vi "9211_UI.vi"(8 "error in (no error)":errorcluster, 11 "Node Ptr":T1 format="%.0x") -> (0 "error out":errorcluster)   [LabVIEW 2019, in "Modules.lvlib" / "9211.lvclass"]
uses:
  9211.lvclass
  <vilib>/NI VeriStand/Custom Device API/Custom Device Item Ref.ctl
  RSI Module/SubPanel Command.ctl
  C:/Users/nitest/Desktop/Git 2019/niveristand-scan-engine-module-libraries/Source/RSI Module/RSI Module.lvclass
  9211.lvclass/9211.ctl
  RSI Module/RSI Module.lvclass
  <vilib>/NI VeriStand/Custom Device API/Custom Device API.lvlib
panel:
  out "_TCTypelabel":string="Thermocouple Type"
  out "_MeasUnitsLabel":string="Measurement Units" caption="MeasUnitsLabel"
  out "_Chan3Label":string="Channel 3"
  out "_Chan2Label":string="Channel 2"
  out "_Chan1Label":string="Channel 1"
  out "_Chan0Label":string="Channel 0"
  in  "Thermocouple Type 3":u8(ring) items=["J", "K", "T", "E", "R", "S", "N", "B"]
  in  "Thermocouple Type 2":u8(ring) items=["J", "K", "T", "E", "R", "S", "N", "B"]
  in  "Thermocouple Type 1":u8(ring) items=["J", "K", "T", "E", "R", "S", "N", "B"]
  in  "Thermocouple Type 0":u8(ring) items=["J", "K", "T", "E", "R", "S", "N", "B"]
  in  "Degree Range AI3":u8(ring)=2 items=["Raw Volts", "Degrees Kelvin", "Degrees Celsius", "Degrees Fahrenheit", "Degrees Rankine"]
  in  "Degree Range AI2":u8(ring)=2 items=["Raw Volts", "Degrees Kelvin", "Degrees Celsius", "Degrees Fahrenheit", "Degrees Rankine"]
  in  "Degree Range AI1":u8(ring)=2 items=["Raw Volts", "Degrees Kelvin", "Degrees Celsius", "Degrees Fahrenheit", "Degrees Rankine"]
  in  "Degree Range AI0":u8(ring)=2 items=["Raw Volts", "Degrees Kelvin", "Degrees Celsius", "Degrees Fahrenheit", "Degrees Rankine"]
  in  "SubPanel Event":refnum<user-event>
  in  "Header":cluster{"Section Name":string}={"Section Name"="NI 9205 Settings"}
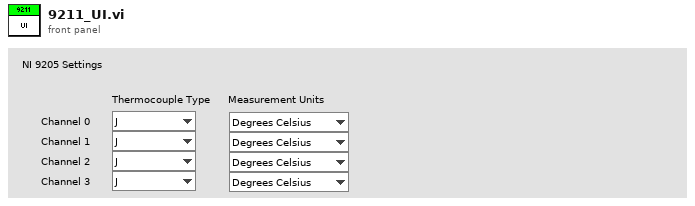
[diagram p1: front panel]
types:
  T1 = typedef "Custom Device API.lvlib/Custom Device Item Ref.ctl" = u64
  T2 = typedef "Modules.lvlib/RSI Module.lvclass/Module Models.ctl" = enum16{"Empty", "NI 9201", "NI 9203", "NI 9205", "NI 9206", "NI 9207", "NI 9208", "NI 9209", "NI 9210", "NI 9211", "NI 9212", "NI 9213", "NI 9214", "NI 9215", "NI 9216", "NI 9217", "NI 9219", "NI 9220", "NI 9221", "NI 9222", "NI 9223", "NI 9224", "NI 9225", "NI 9226", "NI 9227", "NI 9228", "NI 9229", "NI 9233", "NI 9234", "NI 9235", "NI 9236", "NI 9237", "NI 9239", "NI 9242", "NI 9244", "NI 9253", "NI 9263", "NI 9264", "NI 9265", "NI 9266", "NI 9269", "NI 9344", "NI 9350", "NI 9375", "NI 9401", "NI 9402", "NI 9403", "NI 9411", "NI 9421", "NI 9422", "NI 9423", "NI 9425", "NI 9426", "NI 9435", "NI 9436", "NI 9437", "NI 9472", "NI 9474", "NI 9475", "NI 9476", "NI 9477", "NI 9478", "NI 9481", "NI 9482", "NI 9485"}
  T3 = cluster{"Degree range":u32, "Thermocouple type":u32}[]
  T4 = cluster{"Degree range":u32, "Thermocouple type":u32}
  T5 = typedef "Modules.lvlib/RSI Module.lvclass/SubPanel Command.ctl" = enum16{"Stop"}
  T6 = cluster{"Degree Range AI0":u8, "Thermocouple Type 0":u8}
  T7 = cluster{"Degree Range AI1":u8, "Thermocouple Type 1":u8}
  T8 = cluster{"Degree Range AI2":u8, "Thermocouple Type 2":u8}
  T9 = cluster{"Degree Range AI3":u8, "Thermocouple Type 3":u8}
  T10 = cluster{"Degree Range AI3":u8, "Thermocouple Type 3":u8}[]
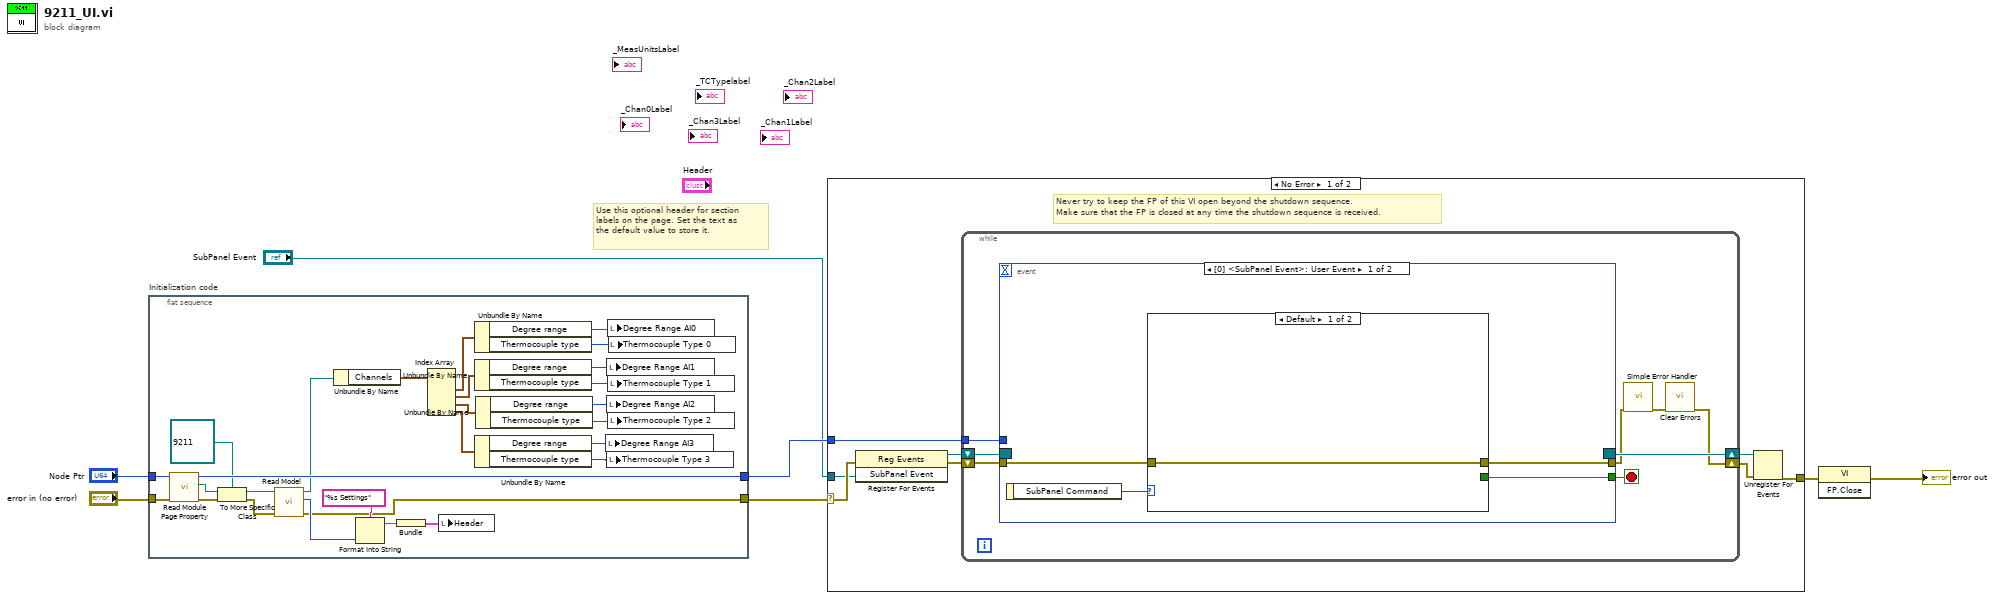
[diagram p0: block diagram]
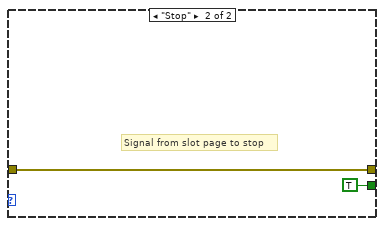
[diagram p2: hidden frame]
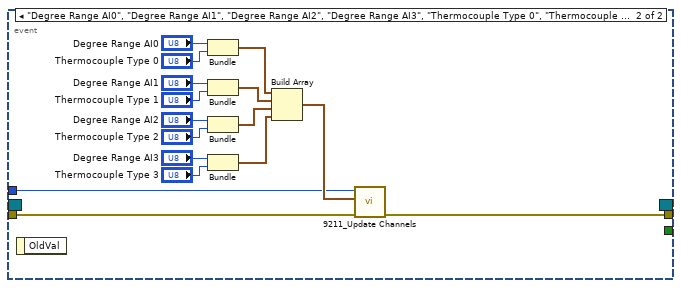
[diagram p3: hidden frame]
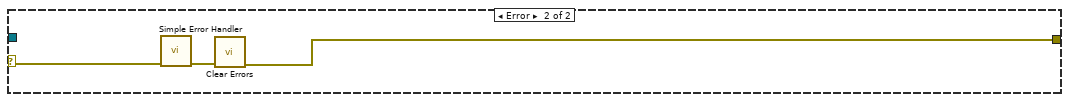
[diagram p4: hidden frame]
diagram:
  # "Use this optional header for section labels on the page. Set the text as the default value to store it."
  n1 = flat-sequence "Initialization code" {
    tunnel: "error in (no error)" -> [w33]
    tunnel: "Node Ptr" -> [w34]
    tunnel: [w21] -> w1
    tunnel: [w32] -> w4
    frame #0 {
      n2 = call "Read Module Page Property.vi"("error in (no error)"=w33, "Node Ptr In"=w34) -> ("error out"=w31:errorcluster, "RSI Module"=w29:refnum<class "RSI Module.lvclass">, "Node Ptr Out"=w32:T1)  [unwired: 7 in]
      n3 = To More Specific Class(target class=refnum<class "9211.lvclass"> refnum ("9205 in"), reference=w29, error in=w31) -> (specific class reference=w28:refnum<class "9211.lvclass">, error out=w27:errorcluster)
      n4 = call "Read Model.vi"("error in (no error)"=w27, "RSI Module in"=w28) -> ("error out"=w21:errorcluster, "Model"=w25:T2, "RSI Module out"=w22:refnum<class "9211.lvclass">)  [unwired: 7 in]
      n5 = Unbundle By Name(w22) -> ("Channels"=w20:T3)
      n6 = Format Into String(format string="%s Settings", w25) -> (resulting string=w23:string)  [unwired: 2 in, 1 out]
      n7 = Bundle(w23) -> (w26:cluster{string})  [unwired: 1 in]
      n8 = Index Array(array=w20) -> (element #1=w17:T4, element #2=w16:T4, element #3=w15:T4, element #4=w14:T4)  [unwired: 4 in]
      n9 = local write "Header"(w26) -> ()
      n10 = Unbundle By Name(w17) -> ("Degree range"=w19:u32, "Thermocouple type"=w18:u32)
      n11 = Unbundle By Name(w16) -> ("Degree range"=w13:u32, "Thermocouple type"=w12:u32)
      n12 = Unbundle By Name(w14) -> ("Degree range"=w9:u32, "Thermocouple type"=w8:u32)
      n13 = Unbundle By Name(w15) -> ("Degree range"=w11:u32, "Thermocouple type"=w10:u32)
      n14 = local write "Degree Range AI3"(w9) -> ()
      n15 = local write "Degree Range AI1"(w13) -> ()
      n16 = local write "Degree Range AI2"(w11) -> ()
      n17 = local write "Thermocouple Type 3"(w8) -> ()
      n18 = local write "Degree Range AI0"(w19) -> ()
      n19 = local write "Thermocouple Type 1"(w12) -> ()
      n20 = local write "Thermocouple Type 2"(w10) -> ()
      n21 = local write "Thermocouple Type 0"(w18) -> ()
    }
  }
  n22 = case shown="No Error" w1 {
    selector: w1 -> [w36 w76]
    tunnel: [w40 w74] -> w7
    tunnel: w4 -> [w37 _]
    tunnel: "SubPanel Event" -> [w35 _]
    frame No Error {
      # "Never try to keep the FP of this VI open beyond the shutdown sequence.\nMake sure that the FP is closed at any time the shutdown sequence is received."
      n23 = register-events(error in=w36, w35) -> (reference out=w38:refnum<event-registration>, error out=w39:errorcluster)  [unwired: 1 in]
      n24 = while {
        tunnel: w37 -> [w46]
        shift-right: [w43] -> w41
        shift-left: w39 -> [w49]
        shift-right: [w50] -> w42
        shift-left: w38 -> [w48]
        stop <- w47 stop-if-true
        n25 = event shown="[0] <SubPanel Event>: User Event" {
          selector: w48 -> [_ _]
          dyn-events: [_ _] -> w50
          timeout: _ -> [_ _]
          tunnel: w49 -> [w53 w60]
          tunnel: [w52 _] -> w47
          tunnel: [w51 w61] -> w45
          tunnel: w46 -> [_ w58]
          event User Event {
            n26 = event-data() -> ("SubPanel Command"=w54:T5)  [unwired: 1 out]
            n27 = case shown="Default" w54 {
              tunnel: w53 -> [w55 w56]
              tunnel: [w55 w56] -> w51
              tunnel: [_ TRUE] -> w52
              frame Default {
              }
              frame "Stop" {
                # "Signal from slot page to stop"
              }
            }
          }
          event "Degree Range AI0", "Degree Range AI1", "Degree Range AI2", "Degree Range AI3", "Thermocouple Type 0", "Thermocouple Type 1", "Thermocouple Type 2", "Thermocouple Type 3": Value Change {
            n28 = event-data() -> ()  [unwired: 2 out]
            n29 = Bundle("Degree Range AI0"="Degree Range AI0", "Thermocouple Type 0"="Thermocouple Type 0") -> (w71:T6)  [unwired: 1 in]
            n30 = Bundle("Degree Range AI1"="Degree Range AI1", "Thermocouple Type 1"="Thermocouple Type 1") -> (w64:T7)  [unwired: 1 in]
            n31 = Bundle("Degree Range AI2"="Degree Range AI2", "Thermocouple Type 2"="Thermocouple Type 2") -> (w63:T8)  [unwired: 1 in]
            n32 = Bundle("Degree Range AI3"="Degree Range AI3", "Thermocouple Type 3"="Thermocouple Type 3") -> (w62:T9)  [unwired: 1 in]
            n33 = Build Array(w71, w64, w63, w62) -> (w59:T10)
            n34 = call "9211_Update Channels.vi"("error in"=w60, "Channels"=w59, "Node Ptr in"=w58) -> ("error out"=w61:errorcluster)  [unwired: 7 in, 1 out]
          }
        }
        n35 = call <vilib>:"Simple Error Handler.vi"("error in (no error)"=w45) -> ("error out"=w44:errorcluster)  [unwired: 1 in, 7 out]
        n36 = call <vilib>:"Clear Errors.vi"("error in (no error)"=w44) -> ("error out"=w43:errorcluster)  [unwired: 1 in, 5 out]
      }
      n37 = Unregister For Events(event registration refnum=w42, error in=w41) -> (error out=w40:errorcluster)
    }
    frame Error {
      n38 = call <vilib>:"Simple Error Handler.vi"("error in (no error)"=w76) -> ("error out"=w75:errorcluster)  [unwired: 1 in, 7 out]
      n39 = call <vilib>:"Clear Errors.vi"("error in (no error)"=w75) -> ("error out"=w74:errorcluster)  [unwired: 1 in, 5 out]
    }
  }
  n40 = invoke class="VI" method="FP.Close"(error in=w7) -> (error out=→"error out":errorcluster)  [unwired: 2 in, 2 out]
